vi "NIDCPower_channel_ganging - close.vi"(8 "error in (no error)":errorcluster, 11 "Ganged Session In":T1) -> (0 "error out":errorcluster)   [LabVIEW 2024]
uses:
  ctl/NIDCPower_channel_ganging - ctl - ganged session.ctl
  ctl/NIDCPower_channel_ganging - ctl - ganged config.ctl
  ctl/NIDCPower_channel_ganging - ctl - channel mode.ctl
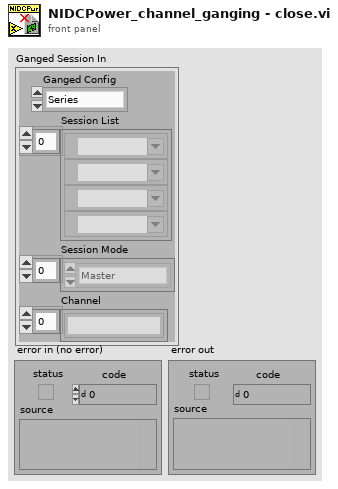
[diagram p1: front panel]
types:
  T1 = typedef "NIDCPower_channel_ganging - ctl - ganged session.ctl" = cluster{"Ganged Config":T2, "Session List":refnum<k15>[], "Session Mode":T3[], "Channel":string[]}
  T2 = typedef "NIDCPower_channel_ganging - ctl - ganged config.ctl" = enum32{"Series", "Parallel", "Manual"}
  T3 = typedef "NIDCPower_channel_ganging - ctl - channel mode.ctl" = enum32{"Master", "Slave", "Slave - Inverted"}
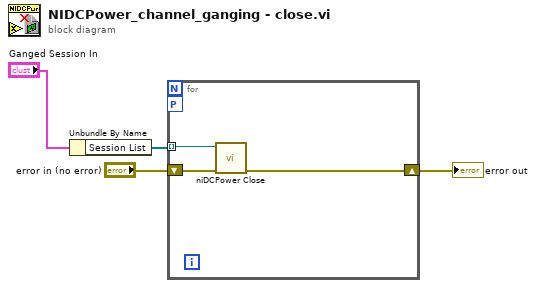
[diagram p0: block diagram]
diagram:
  n1 = Unbundle By Name("Ganged Session In") -> ("Session List"=w2:refnum<k15>[])
  n2 = for {
    shift-right: [w5] -> w3
    shift-left: "error in (no error)" -> [w7]
    tunnel: w2 -> [w6] mode=indexing
    workers-P: _ -> [_]
    n3 = call <instrlib>:"niDCPower Close.vi"("error in (no error)"=w7, "instrument handle"=w6) -> ("error out"=w5:errorcluster)  [unwired: 9 in]
  }
  "error out" <- w3
